vi "get controller name.vi"(8 "error in (no error)":errorcluster, 10 "controller_name":T1, 11 "id":i32) -> (0 "error out":errorcluster, 2 "controller_name out":T1, 3 "function return":i32)   [LabVIEW 2012, in "libximc.lvlib"]
doc: "result_t XIMC_API get_controller_name (device_t id, controller_name_t* controller_name);"
uses:
  libximc.lvlib
  libximc.dll
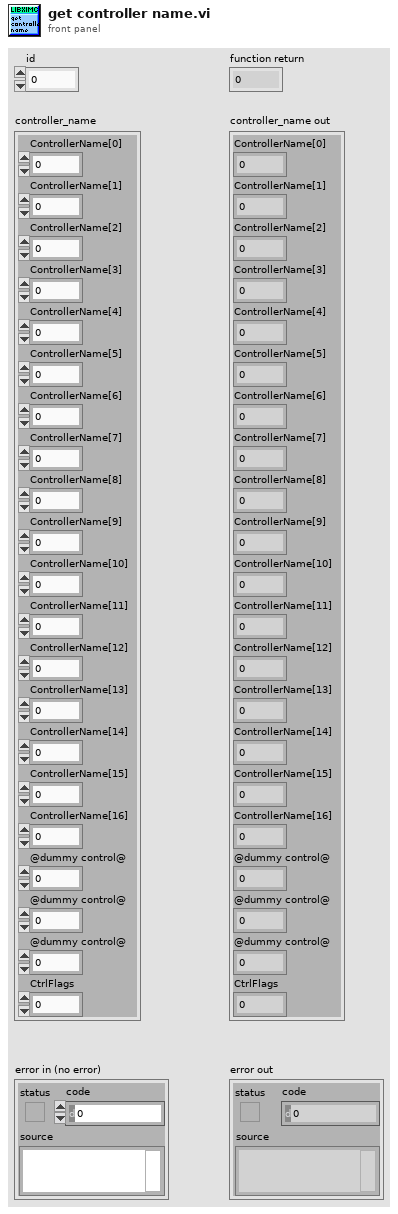
[diagram p1: front panel]
types:
  T1 = cluster{"ControllerName[0]":i8, "ControllerName[1]":i8, "ControllerName[2]":i8, "ControllerName[3]":i8, "ControllerName[4]":i8, "ControllerName[5]":i8, "ControllerName[6]":i8, "ControllerName[7]":i8, "ControllerName[8]":i8, "ControllerName[9]":i8, "ControllerName[10]":i8, "ControllerName[11]":i8, "ControllerName[12]":i8, "ControllerName[13]":i8, "ControllerName[14]":i8, "ControllerName[15]":i8, "ControllerName[16]":i8, "@dummy control@":i8, "@dummy control@":i8, "@dummy control@":i8, "CtrlFlags":u32}
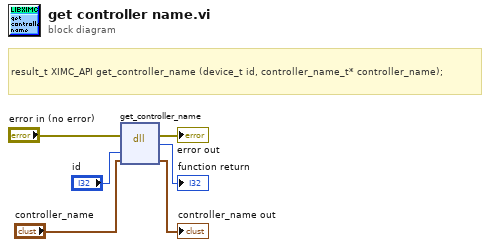
[diagram p0: block diagram]
diagram:
  # "result_t XIMC_API get_controller_name (device_t id, controller_name_t* controller_name);"
  n1 = dll-call lib="C:/Users/Stepan/Downloads/labview_2.9.11_testgen_thread/libximc.*" fn="get_controller_name"(error in="error in (no error)", "id"="id", "controller_name"="controller_name") -> (error out=→"error out":errorcluster, →"function return":i32, "controller_name"=→"controller_name out":T1)  [unwired: 3 in, 1 out]
